vi "File_Module.vi"(7 "Command":T2, 8 "error in (no error)":errorcluster, 9 "All Data":T1={"t(sec)"=1.0, "cycle"=1.0, "DA1(volt)"=1.0, "V1(volt)"=0.0, "V2(volt)"=0.0} {"V2(volt)" format="%.3f"; "cycle" format="%#.3g"; "V1(volt)" format="%.3f"; "DA1(volt)" format="%.3f"; "t(sec)" format="%.1f"}) -> (0 "error out":errorcluster, 2 "selected path":path)   [LabVIEW 2017]
uses:
  File_Module Control.ctl
  Magnitudes Medidas DAC Control.ctl
panel:
  out "Array":string[](array[string])
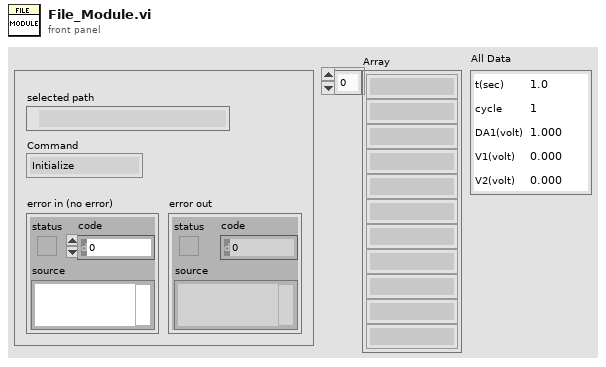
[diagram p1: front panel]
types:
  T1 = typedef "Magnitudes Medidas DAC Control.ctl" = cluster{"t(sec)":dbl, "cycle":dbl, "DA1(volt)":dbl, "V1(volt)":dbl, "V2(volt)":dbl}
  T2 = typedef "File_Module Control.ctl" = enum16{"Initialize", "Save Head", "Save Data", "Shutdown"}
  T3 = enum16{"open", "replace", "create", "open or create", "replace or create", "replace or create with confirmation"}
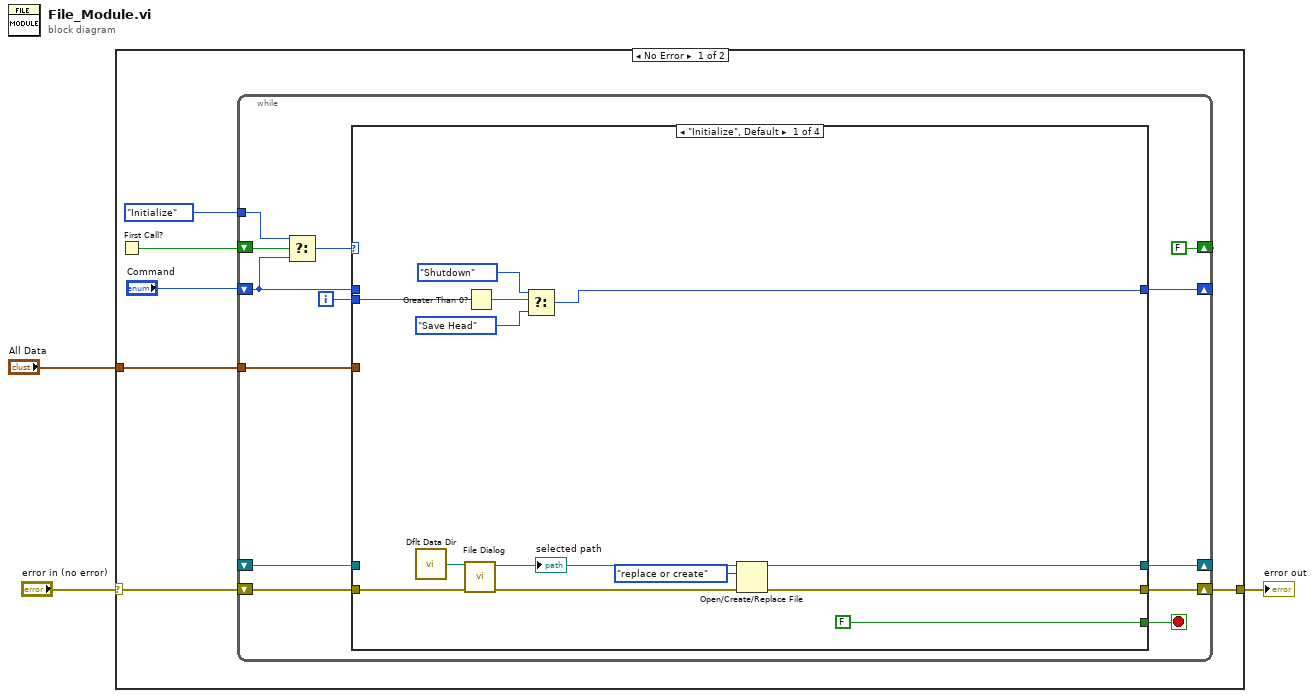
[diagram p0: block diagram]
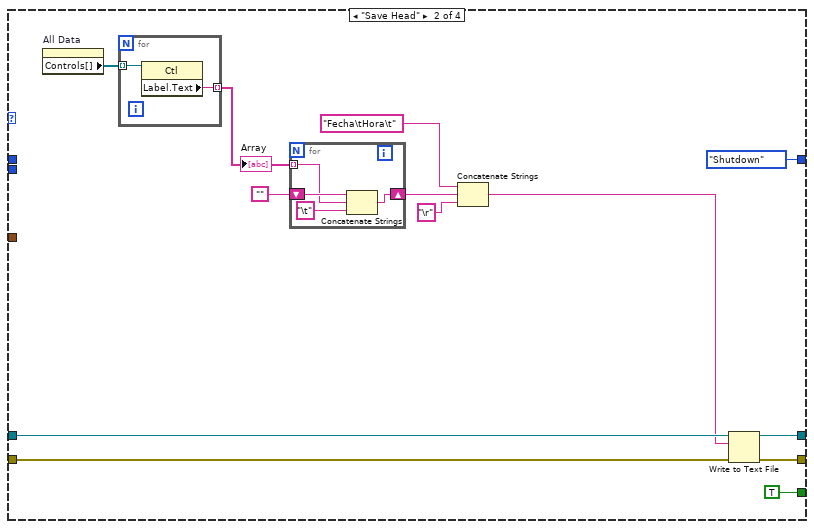
[diagram p2: hidden frame]
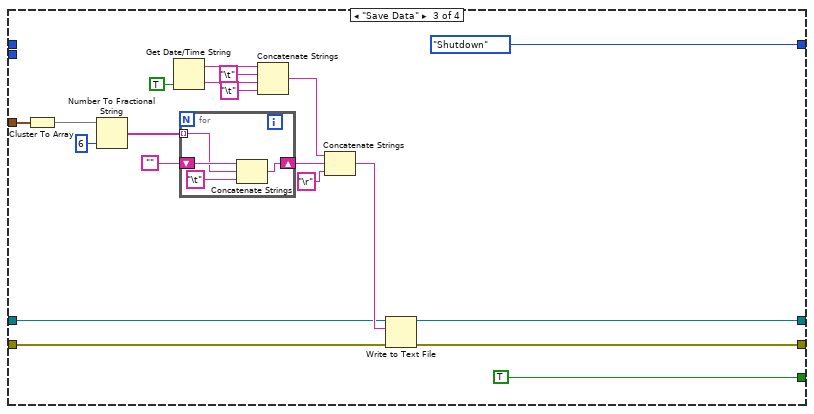
[diagram p3: hidden frame]
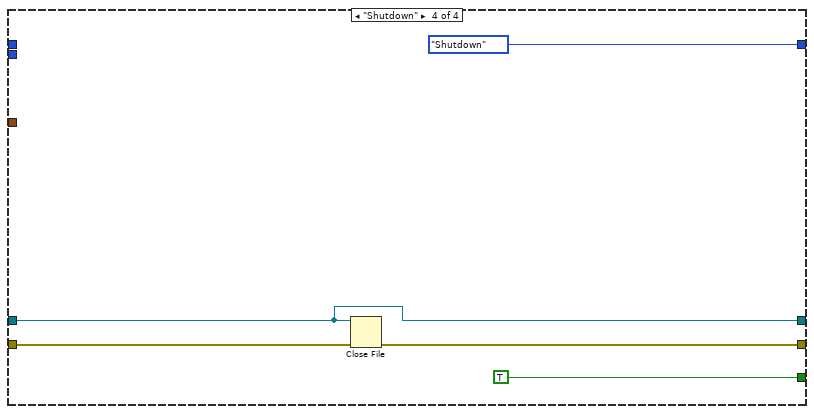
[diagram p4: hidden frame]
diagram:
  n1 = case shown="No Error" "error in (no error)" {
    selector: "error in (no error)" -> [w7 w84]
    tunnel: [w6 w84] -> w2
    tunnel: "All Data" -> [w4 _]
    frame No Error {
      n2 = First Call?() -> (First Call?: T/F=w9:bool)
      n3 = while {
        shift-right: [w14] -> _
        shift-left: "Command" -> [w15]
        shift-right: [w17] -> w6
        shift-left: w7 -> [w18]
        shift-right: [FALSE ("First Call?: T/F")] -> _
        shift-left: w9 -> [w22]
        tunnel: File_Module_Control."Initialize" ("t") -> [w21]
        shift-right: [w11] -> _
        shift-left: _ -> [w12]
        tunnel: w4 -> [w10]
        i -> [w13]
        stop <- w19 stop-if-true
        n4 = Select(t=w21, s=w22, f=w15) -> (s? t:f=w20:T2)
        n5 = case shown="\"Initialize\", Default" w20 {
          tunnel: [FALSE TRUE TRUE TRUE] -> w19
          tunnel: w18 -> [w28 w44 w68 w81]
          tunnel: [w24 w43 w67 w80] -> w17
          tunnel: w15 -> [_ _ _ _]
          tunnel: [w34 File_Module_Control."Shutdown" ("t") File_Module_Control."Shutdown" File_Module_Control."Shutdown"] -> w14
          tunnel: w13 -> [w32 _ _ _]
          tunnel: w12 -> [_ w46 w64 w79]
          tunnel: [w23 w45 w66 w79] -> w11
          tunnel: w10 -> [_ _ w69 _]
          frame "Initialize", Default {
            n6 = call <vilib>:"Dflt Data Dir.vi"() -> ("App:Default Data Directory"=w29:path)
            n7 = call "File Dialog"("start path"=w29, "error in"=w28) -> ("selected path"=w26:path, "error out"=w25:errorcluster)  [unwired: 10 in, 2 out]
            "selected path" <- w26
            n8 = Greater Than 0?(x=w32) -> (x > 0?=w31:bool)
            n9 = Select(t=File_Module_Control."Shutdown", s=w31, f=File_Module_Control."Save Head" ("t")) -> (s? t:f=w34:T2)
            n10 = Open/Create/Replace File(file path (use dialog)=w26, error in=w25, operation (0:open)=T3."replace or create") -> (refnum out=w23:refnum<file>, error out=w24:errorcluster)  [unwired: 3 in, 1 out]
          }
          frame "Save Head" {
            n11 = property on="All Data" class="Clust (strict)"() -> ("Controls[]"=w42:refnum<vi>[])  [unwired: 2 in, 2 out]
            n12 = for {
              tunnel: w42 -> [w54] mode=indexing
              tunnel: [w53] -> w37 mode=indexing
              n13 = property class="Ctl"(reference=w54) -> ("Label.Text"=w53:string)  [unwired: 1 in, 2 out]
            }
            "Array" <- w37
            n14 = for {
              tunnel: w37 -> [w51] mode=indexing
              shift-right: [w50] -> w41
              shift-left: "" -> [w52]
              n15 = Concatenate Strings(w52, w51, "\t" ("string")) -> (w50:string)
            }
            n16 = Concatenate Strings("Fecha\tHora\t" ("string"), w41, "\r" ("string")) -> (w36:string)
            n17 = Write to Text File(file (use dialog)=w46, text=w36, error in=w44) -> (refnum out=w45:refnum<file>, error out=w43:errorcluster)  [unwired: 1 in, 1 out]
          }
          frame "Save Data" {
            n18 = Cluster To Array(cluster=w69) -> (array=w57:dbl[])
            n19 = Number To Fractional String(number=w57, precision (6)=i16 6) -> (F-format string=w56:string[])  [unwired: 2 in]
            n20 = Get Date/Time String(want seconds? (F)=TRUE) -> (date string=w60:string, time string=w59:string)  [unwired: 2 in]
            n21 = for {
              tunnel: w56 -> [w77] mode=indexing
              shift-right: [w76] -> w72
              shift-left: "" -> [w78]
              n22 = Concatenate Strings(w78, w77, "\t" ("string")) -> (w76:string)
            }
            n23 = Concatenate Strings(w60, "\t" ("string"), w59, "\t" ("string")) -> (w63:string)
            n24 = Concatenate Strings(w63, w72, "\r" ("string")) -> (w65:string)
            n25 = Write to Text File(file (use dialog)=w64, text=w65, error in=w68) -> (refnum out=w66:refnum<file>, error out=w67:errorcluster)  [unwired: 1 in, 1 out]
          }
          frame "Shutdown" {
            n26 = Close File(refnum=w79, error in=w81) -> (error out=w80:errorcluster)  [unwired: 1 out]
          }
        }
      }
    }
    frame Error {
    }
  }
  "error out" <- w2
